vi "Start Acquisition.vi"(8 "error in (no error)":errorcluster) -> (0 "error out":errorcluster, 3 "function return":u32)   [LabVIEW 2018, in "AndorSDK.lvlib"]
doc: "EXPNETTYPE unsigned int WINAPI StartAcquisition(void);"
uses:
  AndorSDK.lvlib
  ATMCD32D.dll
  OwnVIs/AndorOWN.lvlib
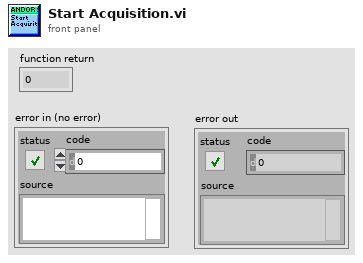
[diagram p1: front panel]
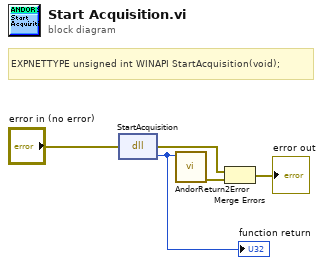
[diagram p0: block diagram]
diagram:
  # "EXPNETTYPE unsigned int WINAPI StartAcquisition(void);"
  n1 = dll-call lib="C:/Users/johan/Downloads/LabVIEW software/LabVIEW software/IX-81 Software/lib/ANDOR/Andor SDK/ATMCD32D.*" fn="StartAcquisition"(error in="error in (no error)") -> (error out=w4:errorcluster, w2:u32)  [unwired: 2 in, 1 out]
  "function return" <- w2
  n2 = call "AndorReturn2Error.vi"("Camera return"=w2) -> ("error out"=w3:errorcluster)  [unwired: 10 in]
  n3 = Merge Errors(w4, w3) -> (→"error out":errorcluster)
